vi "Calib_Ch_setup.vi"(1 "Preston tube diammeter in mm":dbl, 2 "Ch & Spans":T1[](array[typedef]) {"Ch No" min=0 max=7; "low limit (-10V)" min=-10 max=10 format="%.3f"; "high limit (10V)" min=-10 max=10 format="%.3f"}, 3 "Calib filename":path) -> (0 "Output string":string)   [LabVIEW 2013]
uses:
  Controls/TypeCalib.ctl
panel:
  out "length":i32
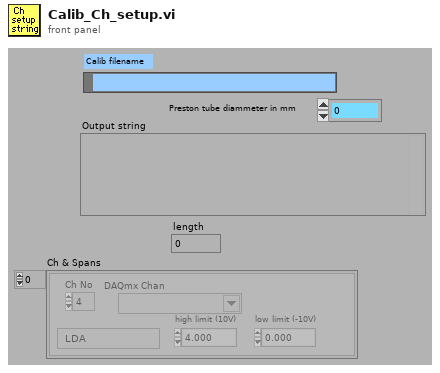
[diagram p1: front panel]
types:
  T1 = typedef "TypeCalib.ctl" = cluster{"high limit (10V)":sgl, "low limit (-10V)":sgl, "Ch No":i16, "Var name":string, "DAQmx Chan":tag}
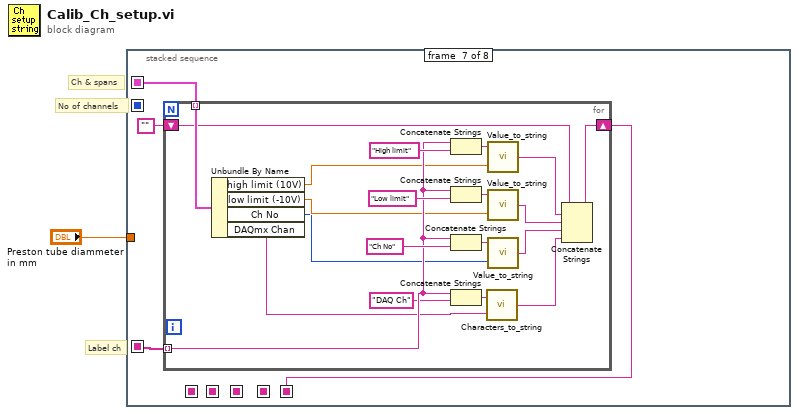
[diagram p0: block diagram]
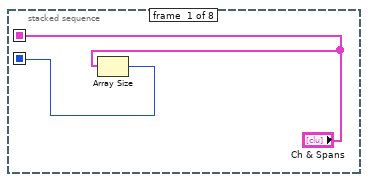
[diagram p2: hidden frame]
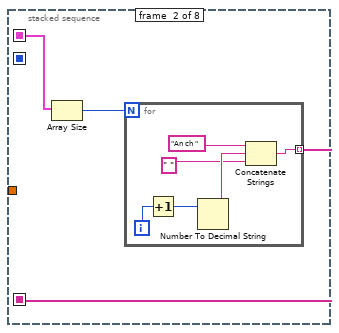
[diagram p3: hidden frame]
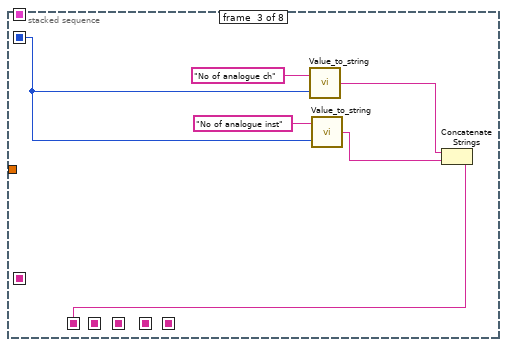
[diagram p4: hidden frame]
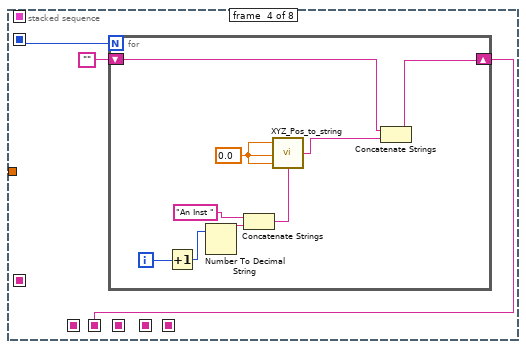
[diagram p5: hidden frame]
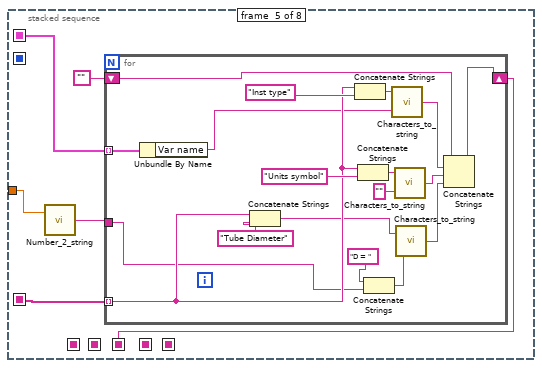
[diagram p6: hidden frame]
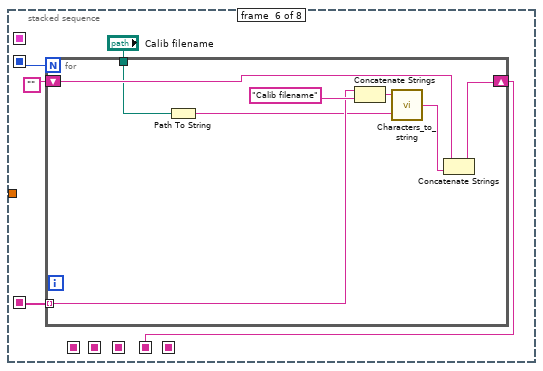
[diagram p7: hidden frame]
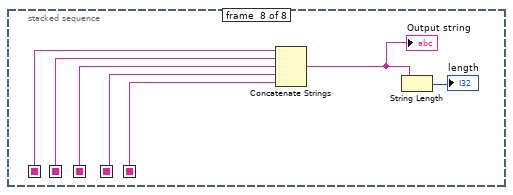
[diagram p8: hidden frame]
diagram:
  # "No of channels"
  # "Ch & spans"
  # "Label ch"
  n1 = stacked-sequence {
    seq-local: [_ _ _ _ w35 _ _ _] -> [_ _ _ _ _ _ _ w98]
    seq-local: [_ _ _ _ _ w57 _ _] -> [_ _ _ _ _ _ _ w97]
    seq-local: [_ _ _ w20 _ _ _ _] -> [_ _ _ _ _ _ _ w96]
    seq-local: [_ w5 _ _ _ _ _ _] -> [_ _ _ _ w34 w58 w70 _]
    seq-local: [_ _ w18 _ _ _ _ _] -> [_ _ _ _ _ _ _ w93]
    seq-local: [_ _ _ _ _ _ w68 _] -> [_ _ _ _ _ _ _ w92]
    seq-local: ["Ch & Spans" _ _ _ _ _ _ _] -> [_ w4 _ _ w33 _ w69 _]
    seq-local: [w3 _ _ _ _ _ _ _] -> [_ _ w16 w19 _ w55 _ _]
    tunnel: "Preston tube diammeter in mm" -> [_ _ _ _ w32 _ _ _]
    frame #0 {
      n2 = Array Size(array="Ch & Spans") -> (size(s)=w3:i32)
    }
    frame #1 {
      n3 = Array Size(array=w4) -> (size(s)=w6:i32)
      n4 = for {
        N: w6 -> [_]
        tunnel: [w8] -> w5 mode=indexing
        i -> [w10]
        n5 = Increment(x=w10) -> (x+1=w9:i32)
        n6 = Number To Decimal String(number=w9) -> (decimal integer string=w12:string)  [unwired: 1 out]
        n7 = Concatenate Strings("An ch ", w12, " ") -> (w8:string)
      }
    }
    frame #2 {
      n8 = call "Value_to_string.vi"("Value"=w16, "Label for value"="No of analogue ch") -> ("Output string"=w17:string)  [unwired: 1 in]
      n9 = call "Value_to_string.vi"("Value"=w16, "Label for value"="No of analogue inst") -> ("Output string"=w14:string)  [unwired: 1 in]
      n10 = Concatenate Strings(w17, w14) -> (w18:string)
    }
    frame #3 {
      n11 = for {
        N: w19 -> [_]
        shift-right: [w29] -> w20
        shift-left: "" -> [w30]
        i -> [w25]
        w22 = 0.0 ("X")
        n12 = Increment(x=w25) -> (x+1=w28:i32)
        n13 = Number To Decimal String(number=w28) -> (decimal integer string=w27:string)  [unwired: 1 out]
        n14 = Concatenate Strings("An Inst ", w27) -> (w23:string)
        n15 = call "XYZ_Pos_to_string.vi"("Position label"=w23, "Z"=w22, "Y"=w22, "X"=w22) -> ("Output string"=w24:string)
        n16 = Concatenate Strings(w30, w24) -> (w29:string)
      }
    }
    frame #4 {
      n17 = call "Number_2_string.vi"("number"=w32) -> ("String"=w31:string)  [unwired: 1 in]
      n18 = for {
        shift-right: [w53] -> w35
        shift-left: "" -> [w54]
        tunnel: w34 -> [w49] mode=indexing
        tunnel: w33 -> [w50] mode=indexing
        tunnel: w31 -> [w46]
        n19 = Unbundle By Name(w50) -> ("Var name"=w43:string)
        n20 = Concatenate Strings(w49, "Tube Diameter") -> (w41:string)
        n21 = Concatenate Strings(w49, "Inst type") -> (w44:string)
        n22 = Concatenate Strings(w49, "Units symbol") -> (w38:string)
        n23 = Concatenate Strings("D = " ("String to match"), w46) -> (w40:string)
        n24 = call "Characters_to_string.vi"("Characters to write"=w43, "Label for characters"=w44) -> ("Output string"=w45:string)
        n25 = call "Characters_to_string.vi"("Characters to write"="", "Label for characters"=w38) -> ("Output string"=w39:string)
        n26 = call "Characters_to_string.vi"("Characters to write"=w40, "Label for characters"=w41) -> ("Output string"=w42:string)
        n27 = Concatenate Strings(w54, w45, w39, w42) -> (w53:string)
      }
    }
    frame #5 {
      n28 = for {
        N: w55 -> [_]
        shift-right: [w66] -> w57
        shift-left: "" -> [w67]
        tunnel: w58 -> [w64] mode=indexing
        tunnel: "Calib filename" -> [w63]
        n29 = Path To String(path=w63) -> (string=w60:string)
        n30 = Concatenate Strings(w64, "Calib filename") -> (w61:string)
        n31 = call "Characters_to_string.vi"("Characters to write"=w60, "Label for characters"=w61) -> ("Output string"=w62:string)
        n32 = Concatenate Strings(w67, w62) -> (w66:string)
      }
    }
    frame #6 {
      n33 = for {
        shift-right: [w84] -> w68
        shift-left: "" -> [w72]
        tunnel: w70 -> [w85] mode=indexing
        tunnel: w69 -> [w77] mode=indexing
        n34 = Unbundle By Name(w77) -> ("high limit (10V)"=w81:sgl, "low limit (-10V)"=w80:sgl, "Ch No"=w79:i16, "DAQmx Chan"=w78:tag)
        n35 = Concatenate Strings(w85, "High limit") -> (w90:string)
        n36 = Concatenate Strings(w85, "Low limit") -> (w89:string)
        n37 = Concatenate Strings(w85, "Ch No") -> (w86:string)
        n38 = Concatenate Strings(w85, "DAQ Ch") -> (w74:string)
        n39 = call "Characters_to_string.vi"("Characters to write"=w78, "Label for characters"=w74) -> ("Output string"=w82:string)
        n40 = call "Value_to_string.vi"("Value"=w81, "Label for value"=w90) -> ("Output string"=w76:string)  [unwired: 1 in]
        n41 = call "Value_to_string.vi"("Value"=w80, "Label for value"=w89) -> ("Output string"=w83:string)  [unwired: 1 in]
        n42 = call "Value_to_string.vi"("Value"=w79, "Label for value"=w86) -> ("Output string"=w75:string)  [unwired: 1 in]
        n43 = Concatenate Strings(w72, w76, w83, w75, w82) -> (w84:string)
      }
    }
    frame #7 {
      n44 = Concatenate Strings(w93, w96, w98, w97, w92) -> (w94:string)
      "Output string" <- w94
      n45 = String Length(string=w94) -> (length=→"length":i32)
    }
  }
